vi "Dashboard.vi"() -> ()   [LabVIEW 2014]
panel:
  in  "Baud Rate":u32=9600
  in  "Serial Port":refnum<visa-resource-name>="COM2"
  out "Lambda 2 R":dbl(slide) scale=0.0..2.0
  out "Lambda 2":dbl(slide) scale=0.0..2.0
  out "Lambda 1 R":dbl(slide) scale=0.0..2.0
  out "Lambda 1":dbl(slide) scale=0.0..2.0
  out "Battery Voltage":dbl(slide) scale=0.0..15.0
  out "Oil Pressure":dbl(knob) scale=0.0..10.0
  out "Air Tenp":dbl(slide) scale=0.0..100.0
  out "Air Box Pressure":dbl(knob) scale=0.0..10.0
  out "Oil Temp":dbl(slide) scale=0.0..100.0
  out "Water Temp":dbl(slide) scale=0.0..100.0
  out "Throttle":dbl(slide) scale=0.0..100.0
  out "RPM":dbl(knob) caption="Gauge 2" scale=0.0..25.0
  out "Speed":dbl(knob) caption="Soeed" scale=0.0..300.0
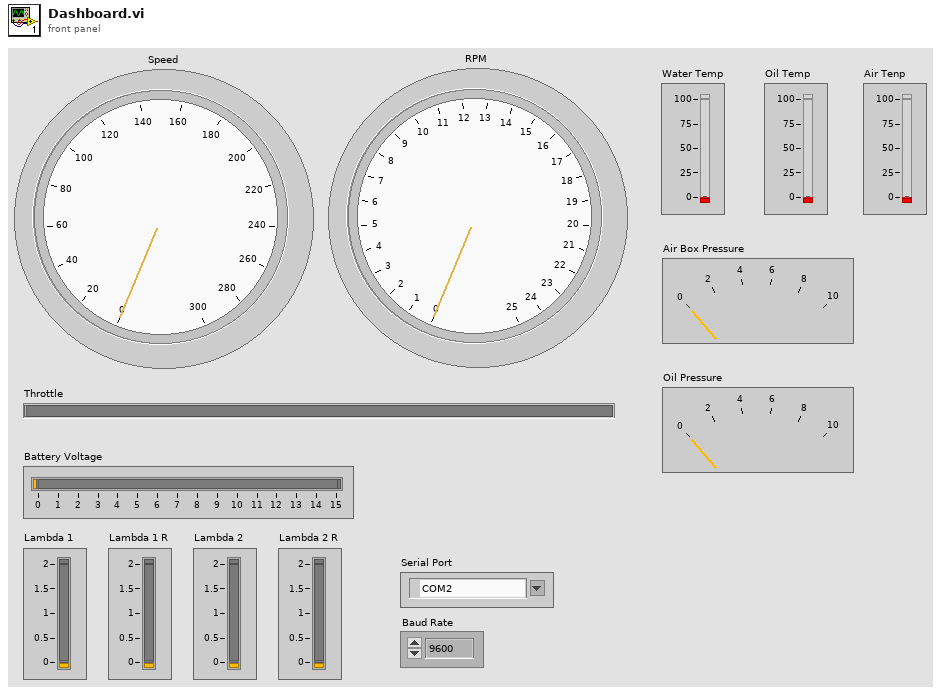
[diagram p1: front panel]
types:
  T1 = typedef "CAR Data Cluster.ctl" = cluster{"revs":dbl[], "rev/min":dbl[], "TPS":dbl[], "map":dbl[], "T H20":dbl[], "T Air":dbl[], "T Oil":dbl[], "Vbb1":dbl[], "Vbb2":dbl[], "Vbb3":dbl[], "Bar0":dbl[], "Lambda 1 AVG":dbl[], "Lambda 1 RAW":dbl[], "Lambda 2 AVG":dbl[], "Lambda 2 RAW":dbl[], "KLambda 1":dbl[], "KLambda 2":dbl[], "Inj Low":dbl[], "Spark 1":dbl[], "Phase Low":dbl[], "Phase High":dbl[], "Speed 1":dbl[], "Speed 2":dbl[], "DTPS+":dbl[], "DTPS-":dbl[], "DECAYINJ(+) - DECAYINJ(-)":dbl[], "DECAYIGN(+) - DECAYIGN(-)":dbl[], "Pot FL":dbl[], "Pot FR":dbl[], "Pot RL":dbl[], "Pot RR":dbl[], "Time":dbl[]}
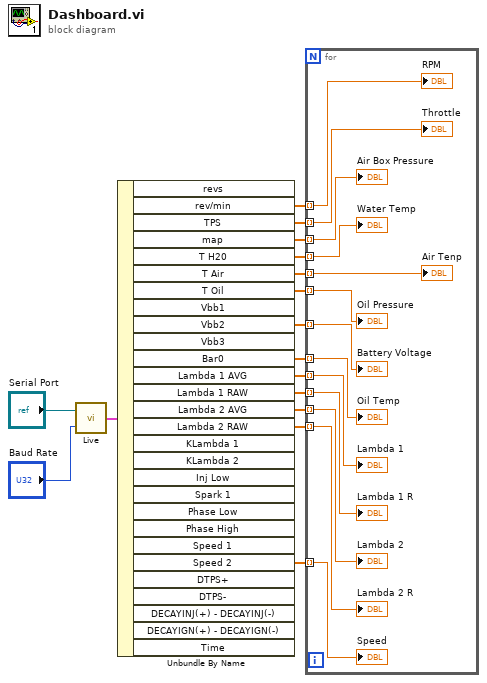
[diagram p0: block diagram]
diagram:
  n1 = call "Live.vi"("baud rate (9600)"="Baud Rate", "VISA Resource (read)"="Serial Port") -> ("CAR DATA"=w16:T1)
  n2 = Unbundle By Name(w16) -> ("rev/min"=w15:dbl[], "TPS"=w14:dbl[], "map"=w13:dbl[], "T H20"=w12:dbl[], "T Air"=w11:dbl[], "T Oil"=w10:dbl[], "Vbb2"=w9:dbl[], "Bar0"=w8:dbl[], "Lambda 1 AVG"=w7:dbl[], "Lambda 1 RAW"=w6:dbl[], "Lambda 2 AVG"=w5:dbl[], "Lambda 2 RAW"=w4:dbl[], "Speed 2"=w3:dbl[])  [unwired: 15 out]
  n3 = for {
    tunnel: w15 -> [w29] mode=indexing
    tunnel: w14 -> [w28] mode=indexing
    tunnel: w13 -> [w27] mode=indexing
    tunnel: w12 -> [w26] mode=indexing
    tunnel: w11 -> [w25] mode=indexing
    tunnel: w10 -> [w24] mode=indexing
    tunnel: w9 -> [w23] mode=indexing
    tunnel: w8 -> [w22] mode=indexing
    tunnel: w7 -> [w21] mode=indexing
    tunnel: w6 -> [w20] mode=indexing
    tunnel: w5 -> [w19] mode=indexing
    tunnel: w4 -> [w18] mode=indexing
    tunnel: w3 -> [w17] mode=indexing
    "Speed" <- w17
    "RPM" <- w29
    "Throttle" <- w28
    "Water Temp" <- w26
    "Oil Temp" <- w22
    "Air Box Pressure" <- w27
    "Air Tenp" <- w25
    "Oil Pressure" <- w24
    "Battery Voltage" <- w23
    "Lambda 1" <- w21
    "Lambda 1 R" <- w20
    "Lambda 2" <- w19
    "Lambda 2 R" <- w18
  }
